vi "stop_program.vi"(0 "Run complete":bool, 1 "Flow Controllers":refnum<visa-resource-name>="COM4", 2 "Fan":refnum<visa-resource-name>="COM4", 3 "Watlows":refnum<visa-resource-name>="COM4", 4 "stop":bool=TRUE, 5 "error in (no error)":errorcluster, 12 "filename":refnum<file>) -> (14 "Reset?":bool=TRUE, 19 "error out":errorcluster)   [LabVIEW 2009]
doc: "Prompts user to confirm quit, then closes datafile and stops vi execution"
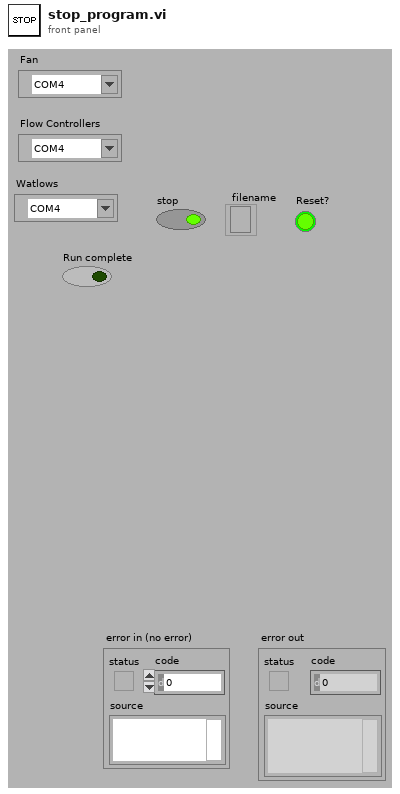
[diagram p1: front panel]
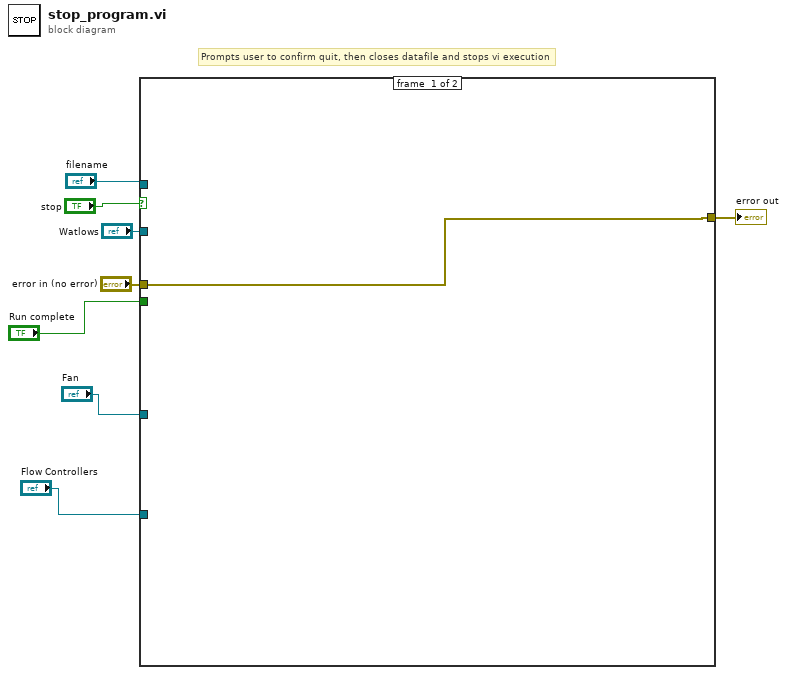
[diagram p0: block diagram]
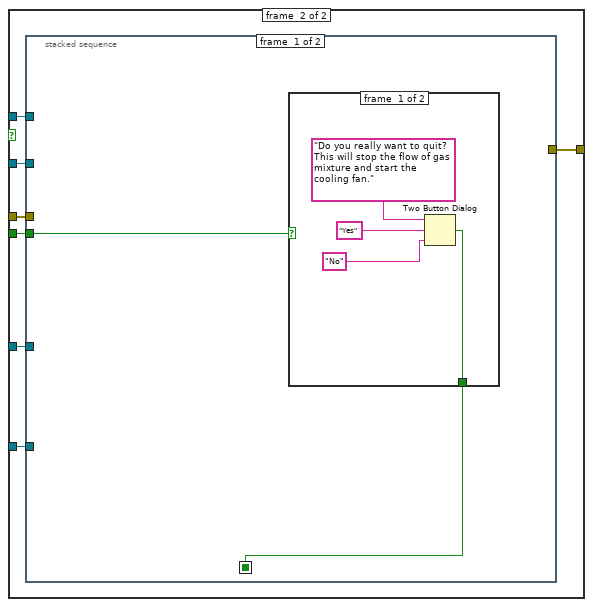
[diagram p2: hidden frame]
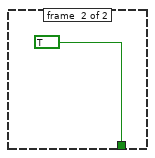
[diagram p3: hidden frame]
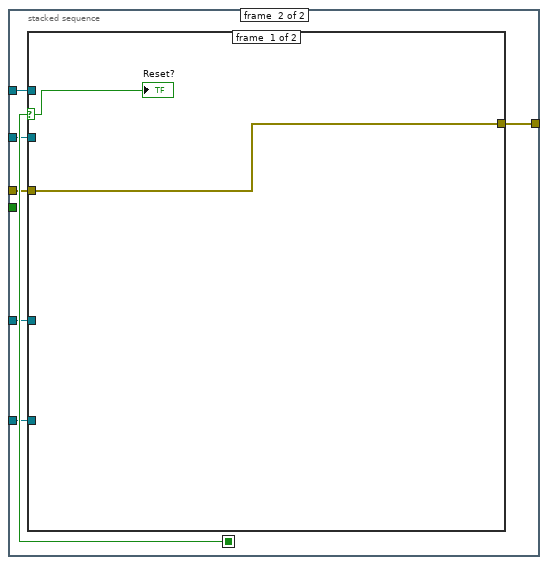
[diagram p4: hidden frame]
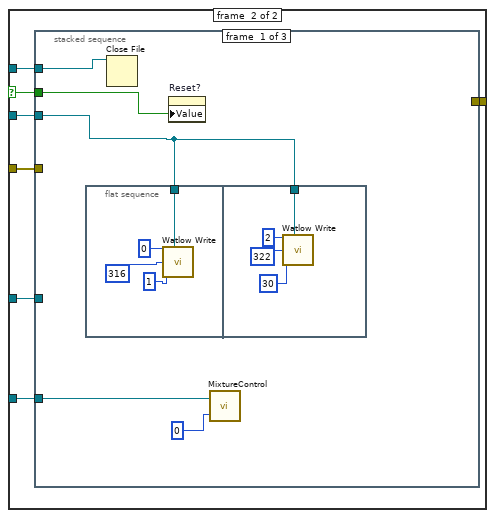
[diagram p5: hidden frame]
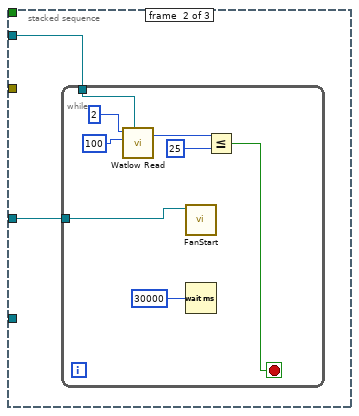
[diagram p6: hidden frame]
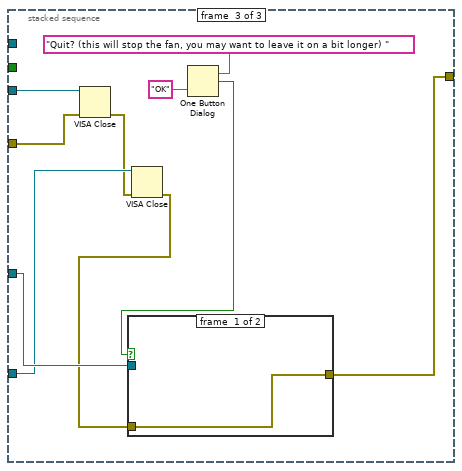
[diagram p7: hidden frame]
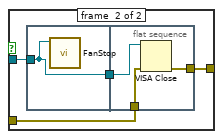
[diagram p8: hidden frame]
diagram:
  # "Prompts user to confirm quit, then closes datafile and stops vi execution"
  n1 = case shown="True" "stop" {
    tunnel: "filename" -> [_ w16]
    tunnel: "error in (no error)" -> [w9 w15]
    tunnel: [w9 w14] -> w5
    tunnel: "Watlows" -> [_ w13]
    tunnel: "Run complete" -> [_ w12]
    tunnel: "Fan" -> [_ w11]
    tunnel: "Flow Controllers" -> [_ w10]
    frame #0 {
    }
    frame #1 {
      n2 = stacked-sequence {
        seq-local: [w18 _] -> [_ w30]
        tunnel: w16 -> [_ w29]
        tunnel: w15 -> [_ w28]
        tunnel: [_ w27] -> w14
        tunnel: w13 -> [_ w26]
        tunnel: w12 -> [w17 _]
        tunnel: w11 -> [_ w25]
        tunnel: w10 -> [_ w24]
        frame #0 {
          n3 = case shown="False" w17 {
            tunnel: [w19 TRUE] -> w18
            frame #0 {
              n4 = Two Button Dialog(message="Do you really want to quit? This will stop the flow of gas mixture and start the cooling fan.", 1:"No", 2:"Yes") -> (T button?=w19:bool)
            }
            frame #1 {
            }
          }
        }
        frame #1 {
          n5 = case shown="True" w30 {
            selector: w30 -> [w32 w38]
            tunnel: w29 -> [_ w39]
            tunnel: w28 -> [w31 w37]
            tunnel: [w31 w36] -> w27
            tunnel: w26 -> [_ w35]
            tunnel: w25 -> [_ w34]
            tunnel: w24 -> [_ w33]
            frame #0 {
              "Reset?" <- w32
            }
            frame #1 {
              n6 = stacked-sequence {
                tunnel: w39 -> [w44 _ _]
                tunnel: w38 -> [w43 _ _]
                tunnel: w37 -> [_ _ w71]
                tunnel: [_ _ w63] -> w36
                tunnel: w35 -> [w42 w54 w72]
                tunnel: w34 -> [_ w53 w68]
                tunnel: w33 -> [w41 _ w67]
                frame #0 {
                  n7 = flat-sequence {
                    tunnel: w42 -> [w45]
                    tunnel: w42 -> [w50]
                    frame #0 {
                      n8 = call "Watlow Write.vi"("Adress"=0, "VISA resource name"=w45, "Register"=u16 316 ("ST-H"), "Parameter"=1) -> ()  [unwired: 1 in, 1 out]
                    }
                    frame #1 {
                      n9 = call "Watlow Write.vi"("Adress"=2, "VISA resource name"=w50, "Register"=u16 322 ("ST-H"), "Parameter"=30) -> ()  [unwired: 1 in, 1 out]
                    }
                  }
                  n10 = Close File(refnum=w44) -> ()  [unwired: 1 in, 2 out]
                  n11 = property on="Reset?" class="Bool (strict)"("Value"=w43) -> ()  [unwired: 2 in, 2 out]
                  n12 = call "MixtureControl.vi"("%CO2"=0, "VISA resource name"=w41) -> ()  [unwired: 1 in]
                }
                frame #1 {
                  n13 = while {
                    tunnel: w54 -> [w59]
                    tunnel: w53 -> [w55]
                    stop <- w56 stop-if-true
                    n14 = call "Watlow Read.vi"("Adress"=2, "Register"=100, "VISA resource name"=w59) -> ("Number"=w57:u32)  [unwired: 1 in, 2 out]
                    n15 = call "FanStart.vi"("VISA resource name"=w55) -> ()  [unwired: 11 in]
                    n16 = Wait (ms)(milliseconds to wait=u32 30000) -> ()  [unwired: 1 out]
                    n17 = Less Or Equal?(x=w57, y=25) -> (x <= y?=w56:bool)
                  }
                }
                frame #2 {
                  n18 = VISA Close(VISA resource name=w72, error in (no error)=w71) -> (error out=w66:errorcluster)
                  n19 = VISA Close(VISA resource name=w67, error in (no error)=w66) -> (error out=w64:errorcluster)
                  n20 = One Button Dialog(message="Quit? (this will stop the fan, you may want to leave it on a bit longer) ", button name ("OK")="OK") -> (true=w70:bool)
                  n21 = case shown="True" w70 {
                    tunnel: w68 -> [_ w75]
                    tunnel: w64 -> [w73 w77]
                    tunnel: [w73 w76] -> w63
                    frame #0 {
                    }
                    frame #1 {
                      n22 = flat-sequence {
                        tunnel: w75 -> [w78]
                        tunnel: [w78] -> w74
                        tunnel: w77 -> [w81]
                        tunnel: [w80] -> w76
                        tunnel: w74 -> [w79]
                        frame #0 {
                          n23 = call "FanStop.vi"("VISA resource name"=w78) -> ()  [unwired: 11 in]
                        }
                        frame #1 {
                          n24 = VISA Close(VISA resource name=w79, error in (no error)=w81) -> (error out=w80:errorcluster)
                        }
                      }
                    }
                  }
                }
              }
            }
          }
        }
      }
    }
  }
  "error out" <- w5
